vi "Page_Info_Write.vi"(6 "ctlReferences":T1, 8 "error in (no error)":errorcluster, 10 "Target filename":string, 11 "AB_Deploy_EXE in":refnum<class "AB_Deploy_EXE.lvclass">) -> (0 "error out":errorcluster, 3 "AB_Deploy_EXE out":refnum<class "AB_Deploy_EXE.lvclass">)   [LabVIEW 2020, in "AB_Deploy_EXE.lvclass"]
uses:
  <vilib>/AppBuilder/AB_Classes/DeployableEXE/AB_Deploy_EXE.lvclass
  <resource>/Framework/Providers/Builds/AppBuilder/AB_UI_Page_Info_References.ctl
  e:/builds/penguin/labview/branches/2020/dev/dist/vi.lib/AppBuilder/AB_Classes/TargetFile/AB_Targetfile.lvclass
  e:/builds/penguin/labview/branches/2020/dev/dist/vi.lib/AppBuilder/AB_Classes/Build/AB_Build.lvclass
  <vilib>/AppBuilder/AB_Classes/DeployableEXE/AB_Deploy_EXE.lvclass/AB_Deploy_EXE.ctl
  <vilib>/AppBuilder/AB_Classes/EXE/AB_EXE.lvclass
  <vilib>/AppBuilder/AB_Classes/Destination/AB_Destination.lvclass
  <vilib>/AppBuilder/AB_Classes/Build/AB_Build.lvclass
  <vilib>/AppBuilder/AB_Classes/TargetFile/AB_Targetfile.lvclass
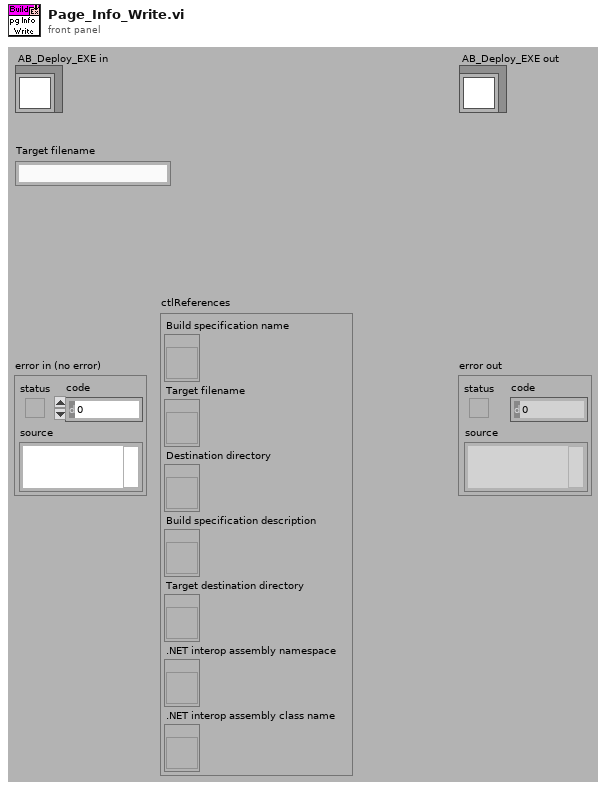
[diagram p1: front panel]
types:
  T1 = typedef "AB_UI_Page_Info_References.ctl" = cluster{"Build specification name":refnum<vi>, "Target filename":refnum<vi>, "Destination directory":refnum<vi>, "Build specification description":refnum<vi>, "Target destination directory":refnum<vi>, ".NET interop assembly namespace":refnum<vi>, ".NET interop assembly class name":refnum<vi>}
  T2 = typedef "AB_Targetfile.ctl" = cluster{"targetfileName":string, "targetfileGUID":string, "enableDebugging":bool, "versionInfo":cluster{"productName":string, "legalCopyright":string, "companyName":string, "internalName":string, "fileDescription":string}, "eng_consolidatedTypeInfo":string, "fastFileFormat":bool, "eng_LEIFBuildData":u32, "versionIndependent":bool}
  T3 = typedef "AB_Build.ctl" = cluster{"buildSpecName":string, "buildSpecDescription":string, "destinations":refnum<class "AB_Destination.lvclass">[], "exclusionOption":T4, "defaultLanguage":string, "supportedLanguages":string[], "excludedDirectories":path[], "buildContext":refnum<vi>, "buildObject":T5, "preview":bool, "programatic":bool, "progressBarEvents":T6, "userLog_Path":path, "preActionID":string, "preAction_Path":path, "postActionID":string, "postAction_Path":path, "eng_checkForBrokenVIs?":bool, "eng_verboseLinkerErrors?":bool, "localDest_Path":path, "targetDest_Path":path, "removeVIObject":u16, "cache":refnum<class "PreviewCache.lvclass">, "use cache":bool, "previewCache_ID":string, "buildCache_ID":string, "eng_TempLocalDest_Path":path, "eng_collectDependencies?":bool, "versionInfo":cluster{"buildVersion":cluster{"major":u16, "minor":u16, "patch":u16, "build":u16}, "autoIncrement":bool}, "eng_enableVIChecksums":bool}
  T4 = typedef "AB_Exclusion_Option.ctl" = cluster{"typedefs":bool, "polymorphicVIs":bool, "unusedLibraryItems":bool, "modifyLibraryFile":bool, "edit-timeDependencies":bool, "inlineVIs":bool, "dependent PPLs":bool, "dependent DLLs":bool}
  T5 = typedef "ItemRef.ctl" = u64
  T6 = typedef "provcom_ProgressBar_Events.ctl" = cluster{"newJob":refnum<user-event>, "newItem":refnum<user-event>, "errorMsg":T7, "cancel":refnum<user-event>}
  T7 = typedef "mxLvBuildError.ctl" = refnum<user-event>
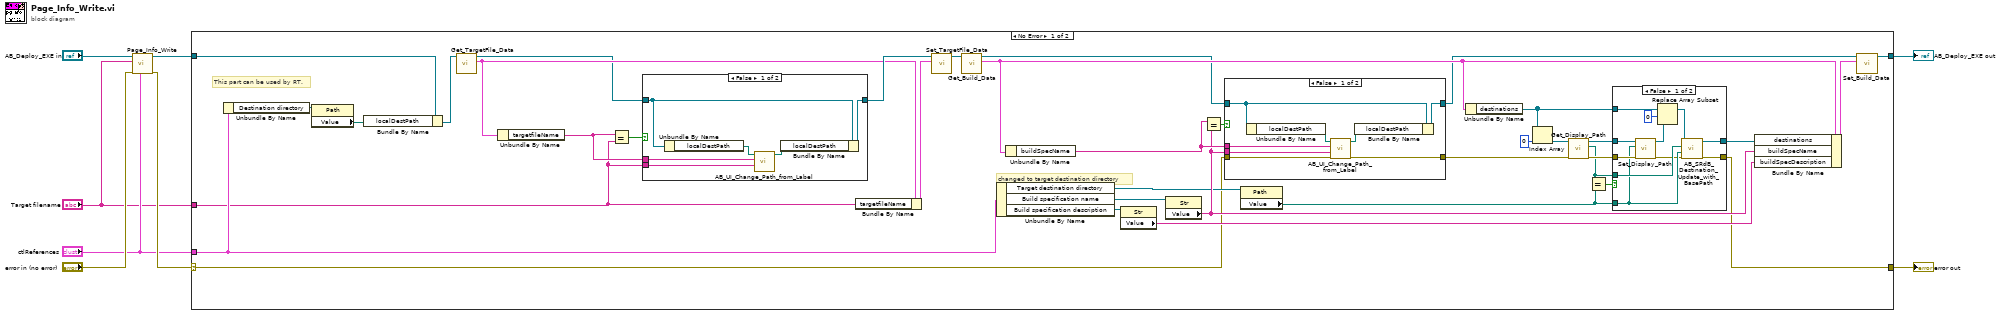
[diagram p0: block diagram]
diagram:
  n1 = call-parent "Page_Info_Write.vi"("ctlReferences"="ctlReferences", "error in (no error)"="error in (no error)", "Target filename"="Target filename", "AB_EXE in"="AB_Deploy_EXE in") -> ("error out"=w3:errorcluster, "AB_EXE out"=w5:refnum<class "AB_Deploy_EXE.lvclass">)  [unwired: 6 in]
  n2 = case shown="No Error" w3 {
    selector: w3 -> [w10 w77]
    tunnel: [w28 w77] -> w8
    tunnel: "ctlReferences" -> [w17 _]
    tunnel: w5 -> [w15 w76]
    tunnel: [w13 w76] -> w7
    tunnel: "Target filename" -> [w9 _]
    frame No Error {
      # "This part can be used by RT."
      # "changed to target destination directory"
      n3 = Unbundle By Name(w17) -> ("Destination directory"=w18:refnum<vi>)
      n4 = property class="Path"(reference=w18) -> ("Value"=w16:path)  [unwired: 1 in, 2 out]
      n5 = Bundle By Name(cluster=w15, "localDestPath"=w16) -> (w14:refnum<class "AB_Deploy_EXE.lvclass">)
      n6 = call <vilib>:"Get_TargetFile_Data.vi"("AB_Targetfile in"=w14) -> ("data"=w23:T2, "AB_Targetfile out"=w11:refnum<class "AB_Deploy_EXE.lvclass">)  [unwired: 8 in, 1 out]
      n7 = Unbundle By Name(w23) -> ("targetfileName"=w12:string)
      n8 = Equal?(x=w12, y=w9) -> (x = y?=w27:bool)
      n9 = case shown="False" w27 {
        tunnel: w9 -> [w49 _]
        tunnel: w12 -> [w50 _]
        tunnel: w11 -> [w48 w52]
        tunnel: [w47 w52] -> w24
        frame False {
          n10 = Unbundle By Name(w48) -> ("localDestPath"=w51:path)
          n11 = call <resource>:"AB_UI_Change_Path_from_Label.vi"("new label"=w49, "old label"=w50, "Path in"=w51) -> ("Path out"=w46:path)  [unwired: 6 in, 2 out]
          n12 = Bundle By Name(cluster=w48, "localDestPath"=w46) -> (w47:refnum<class "AB_Deploy_EXE.lvclass">)
        }
        frame True {
        }
      }
      n13 = Bundle By Name(cluster=w23, "targetfileName"=w9) -> (w25:T2)
      n14 = call <vilib>:"Set_TargetFile_Data.vi"("data"=w25, "AB_Targetfile in"=w24) -> ("AB_Targetfile out"=w26:refnum<class "AB_Deploy_EXE.lvclass">)  [unwired: 8 in, 1 out]
      n15 = call <vilib>:"Get_Build_Data.vi"("Class in"=w26) -> ("data"=w22:T3, "Class out"=w21:refnum<class "AB_Deploy_EXE.lvclass">)  [unwired: 8 in, 1 out]
      n16 = Unbundle By Name(w17) -> ("Target destination directory"=w33:refnum<vi>, "Build specification name"=w45:refnum<vi>, "Build specification description"=w44:refnum<vi>)
      n17 = Unbundle By Name(w22) -> ("buildSpecName"=w41:string)
      n18 = property class="Str"(reference=w44) -> ("Value"=w43:string)  [unwired: 1 in, 2 out]
      n19 = property class="Str"(reference=w45) -> ("Value"=w40:string)  [unwired: 1 in, 2 out]
      n20 = Equal?(x=w41, y=w40) -> (x = y?=w42:bool)
      n21 = case shown="False" w42 {
        tunnel: w40 -> [w72 _]
        tunnel: w41 -> [w73 _]
        tunnel: [w69 w75] -> w31
        tunnel: w10 -> [w70 w75]
        tunnel: w21 -> [w71 w74]
        tunnel: [w66 w74] -> w20
        frame False {
          n22 = Unbundle By Name(w71) -> ("localDestPath"=w68:path)
          n23 = call <resource>:"AB_UI_Change_Path_from_Label.vi"("error in (no error)"=w70, "new label"=w72, "old label"=w73, "Path in"=w68) -> ("error out"=w69:errorcluster, "Path out"=w67:path)  [unwired: 5 in, 1 out]
          n24 = Bundle By Name(cluster=w71, "localDestPath"=w67) -> (w66:refnum<class "AB_Deploy_EXE.lvclass">)
        }
        frame True {
        }
      }
      n25 = property class="Path"(reference=w33) -> ("Value"=w32:path)  [unwired: 1 in, 2 out]
      n26 = Unbundle By Name(w22) -> ("destinations"=w19:refnum<class "AB_Destination.lvclass">[])
      n27 = Index Array(array=w19, index=0) -> (element=w38:refnum<class "AB_Destination.lvclass">)
      n28 = call-dynamic "Get_Display_Path.vi"("error in (no error)"=w31, "AB_Destination in"=w38) -> ("error out"=w36:errorcluster, "displayPath"=w35:path, "AB_Destination out"=w37:refnum<class "AB_Destination.lvclass">)  [unwired: 7 in]
      n29 = Equal?(x=w35, y=w32) -> (x = y?=w34:bool)
      n30 = case shown="False" w34 {
        tunnel: w36 -> [w61 w64]
        tunnel: w32 -> [w60 _]
        tunnel: w35 -> [w63 _]
        tunnel: w37 -> [w62 _]
        tunnel: w19 -> [w58 w65]
        tunnel: [w54 w65] -> w30
        tunnel: [w53 w64] -> w28
        frame False {
          n31 = call-dynamic "Set_Display_Path.vi"("error in (no error)"=w61, "displayPath"=w60, "AB_Destination in"=w62) -> ("error out"=w56:errorcluster, "AB_Destination out"=w59:refnum<class "AB_Destination.lvclass">)  [unwired: 7 in]
          n32 = Replace Array Subset(array=w58, new element=w59, index=0) -> (w57:refnum<class "AB_Destination.lvclass">[])
          n33 = call <resource>:"AB_SRdB_Destination_Update_with_BasePath.vi"("error in (no error)"=w56, "new base path"=w60, "old base path"=w63, "ALL data in"=w57) -> ("error out"=w53:errorcluster, "ALL data out"=w54:refnum<class "AB_Destination.lvclass">[])  [unwired: 6 in]
        }
        frame True {
        }
      }
      n34 = Bundle By Name(cluster=w22, "destinations"=w30, "buildSpecName"=w40, "buildSpecDescription"=w43) -> (w29:T3)
      n35 = call <vilib>:"Set_Build_Data.vi"("data"=w29, "Class in"=w20) -> ("Class out"=w13:refnum<class "AB_Deploy_EXE.lvclass">)  [unwired: 8 in, 1 out]
    }
    frame Error {
    }
  }
  "error out" <- w8
  "AB_Deploy_EXE out" <- w7
